vi "API Tree.vi"   [LabVIEW 2021]
panel:
  # "SEE DIAGRAM\nFOR Hierarchy"
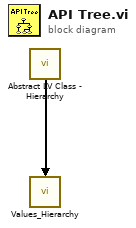
[diagram p0: block diagram]
diagram:
  n1 = call "Abstract LV Class - Hierarchy.vi"() -> ()  [unwired: 12 in]
  n2 = call "Values_Hierarchy.vi"() -> ()  [unwired: 12 in]
